vi "Convert NT Types.vi"(11 "Type in":T1) -> (3 "Type out":u8)   [LabVIEW 2017]
uses:
  <vilib>/Rock Robotics/Network Tables/Field Type.ctl
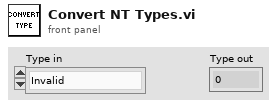
[diagram p1: front panel]
types:
  T1 = typedef "Field Type.ctl" = enum8{"Invalid", "Bool", "Numeric", "String", "Raw", "Boolean Array", "Numeric Array", "String Array", "RPC"}
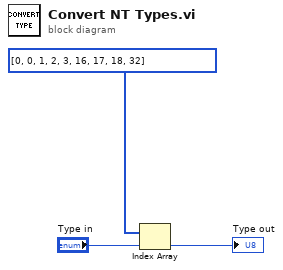
[diagram p0: block diagram]
diagram:
  n1 = Index Array(array=u8[] [0, 0, 1, 2, 3, 16, 17, 18, 32], index="Type in") -> (element=→"Type out":u8)
